vi "Get Sender.vi"(11 "Teardown Msg Strategy in":refnum<class "Teardown Msg Strategy.lvclass">) -> (2 "Sender":refnum<class "Sender.lvclass">)   [LabVIEW 2021, in "jettl.lvlib" / "Teardown Msg Strategy.lvlib" / "Teardown Msg Strategy.lvclass"]
uses:
  Teardown Msg Strategy.lvclass
  Teardown Msg Strategy.lvclass/Teardown Msg Strategy.ctl
  Sender/Sender/Sender.lvclass
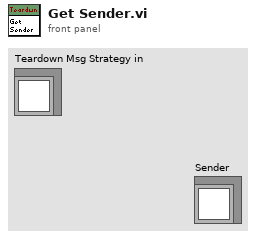
[diagram p1: front panel]
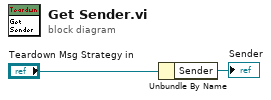
[diagram p0: block diagram]
diagram:
  n1 = Unbundle By Name("Teardown Msg Strategy in") -> ("Sender"=→"Sender":refnum<class "Sender.lvclass">)
